vi "Tosca-Evaluate Input Event.vi"(0 "Progress In":T2, 1 "Event state in":T1, 7 "Term":refnum<class "Termination.lvclass">) -> (3 "Event state out":T1, 4 "Progress Out":T2, 8 "TTL condition true":bool)   [LabVIEW 2020]
uses:
  Typedefs/Tosca-Transition Progress.ctl
  Typedefs/Tosca-Trial Result Enum.ctl
  Typedefs/Tosca-TTL Event State.ctl
  Classes/Termination/Termination.lvclass
  Typedefs/Tosca-Termination Condition Action.ctl
  Classes/Termination/Termination.lvclass/Termination.ctl
  Classes/Termination/Read Input.vi
  Classes/Termination/Read Latency (ms).vi
  Classes/Termination/Read End after (ms).vi
  Classes/Termination/Read Action.vi
  Classes/Termination/Read Next.vi
  Classes/Termination/Read End on rep.vi
  Classes/Termination/Read Nttl.vi
  Classes/Termination/Read Tttl.vi
  Classes/Termination/Read Source.vi
  Classes/Termination/Read Result.vi
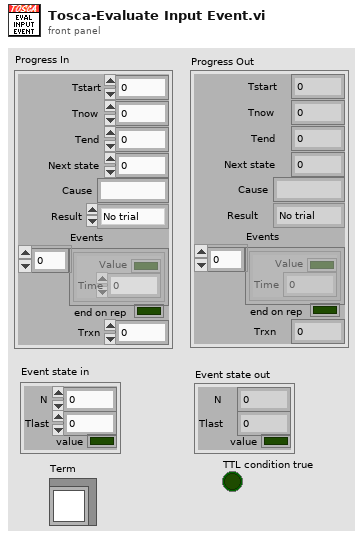
[diagram p1: front panel]
types:
  T1 = typedef "Tosca-TTL Event State.ctl" = cluster{"N":i32, "Tlast":dbl, "value":bool}
  T2 = typedef "Tosca-Transition Progress.ctl" = cluster{"Tstart":u32, "Tnow":u32, "Tend":dbl, "Next state":i32, "Cause":string, "Result":T3, "Events":cluster{"Value":bool, "Time":u32}[], "end on rep":bool, "Trxn":i32}
  T3 = typedef "Tosca-Trial Result Enum.ctl" = enum16{"No trial", "Go", "No go", "Error", "Abort"}
  T4 = typedef "Tosca-Termination Condition Action.ctl" = enum16{"End state", "Complete state", "TTL only"}
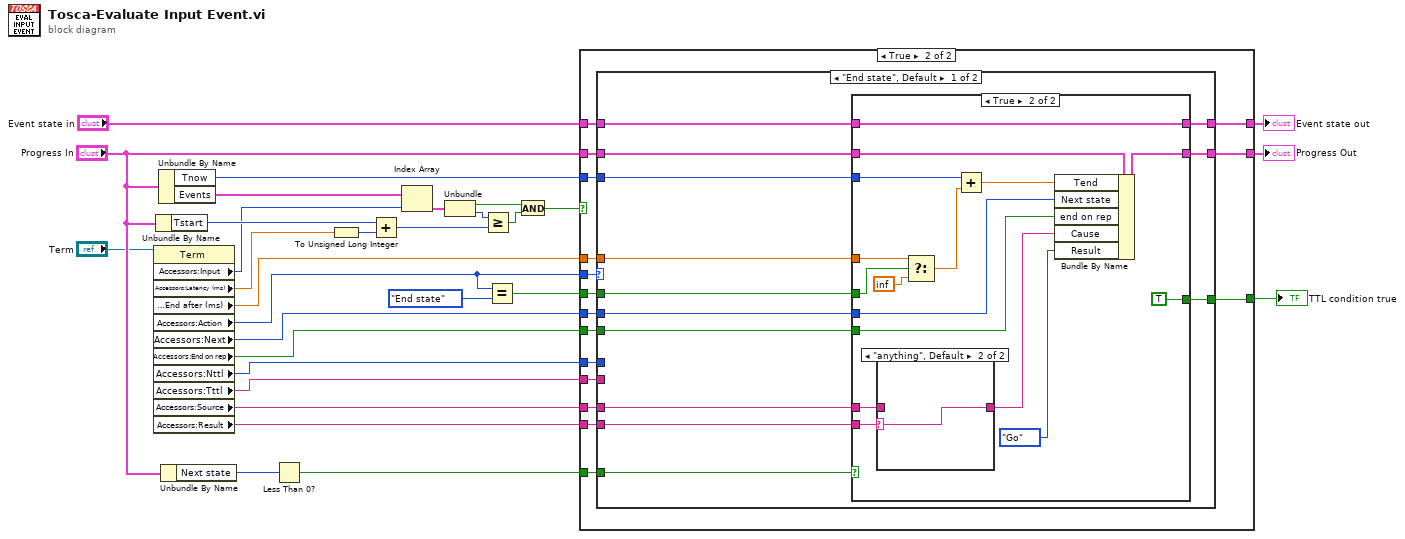
[diagram p0: block diagram]
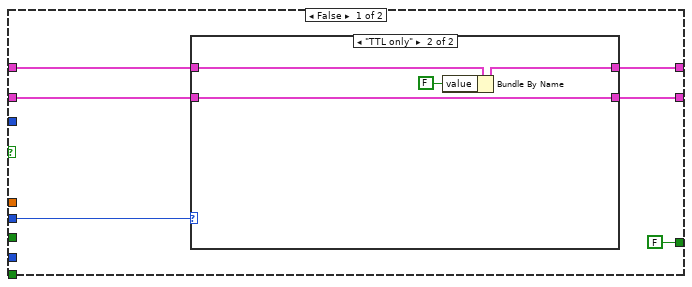
[diagram p2: hidden frame]
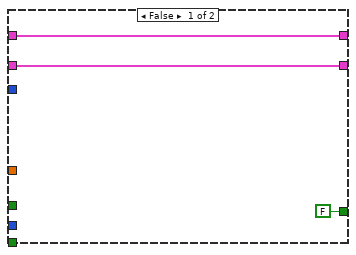
[diagram p4: hidden frame]
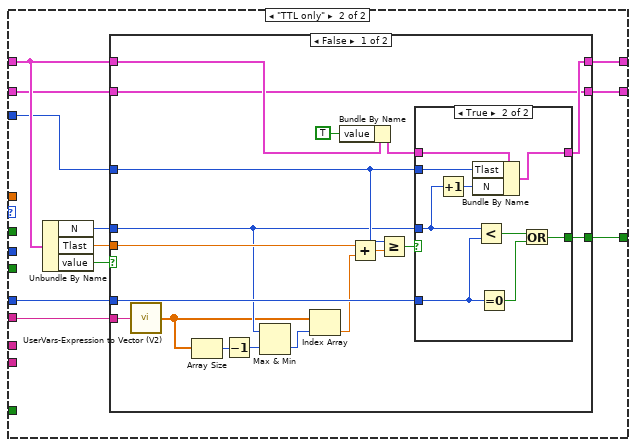
[diagram p6: hidden frame]
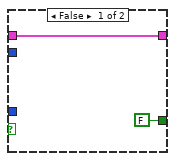
[diagram p7: hidden frame]
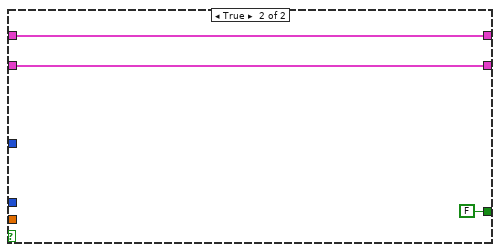
[diagram p8: hidden frame]
diagram:
  n1 = property class="Term"(reference="Term") -> ("Accessors:Input"=w1:i32, "Accessors:Latency (ms)"=w3:dbl, "Accessors:End after (ms)"=w4:dbl, "Accessors:Action"=w5:T4, "Accessors:Next"=w2:i32, "Accessors:End on rep"=w6:bool, "Accessors:Nttl"=w7:i32, "Accessors:Tttl"=w8:string, "Accessors:Source"=w9:string, "Accessors:Result"=w10:string)  [unwired: 1 in, 2 out]
  n2 = Unbundle By Name("Progress In") -> ("Tstart"=w20:u32)
  n3 = Unbundle By Name("Progress In") -> ("Tnow"=w23:u32, "Events"=w27:cluster{"Value":bool, "Time":u32}[])
  n4 = Unbundle By Name("Progress In") -> ("Next state"=w13:i32)
  n5 = Less Than 0?(x=w13) -> (x < 0?=w12:bool)
  n6 = To Unsigned Long Integer(number=w3) -> (unsigned 32bit integer=w21:u32)
  n7 = Add(x=w20, y=w21) -> (x+y=w22:u32)
  n8 = Index Array(array=w27, index=w1) -> (element=w30:cluster{"Value":bool, "Time":u32})
  n9 = Unbundle(w30) -> ("Value"=w26:bool, "Time"=w25:u32)
  n10 = Greater Or Equal?(x=w25, y=w22) -> (x >= y?=w28:bool)
  n11 = Equal?(x=w5, y=Tosca-Termination_Condition_Action."End state") -> (x = y?=w19:bool)
  n12 = And(x=w26, y=w28) -> (x .and. y?=w29:bool)
  n13 = case shown="True" w29 {
    tunnel: w4 -> [_ w57]
    tunnel: w19 -> [_ w58]
    tunnel: "Progress In" -> [w32 w56]
    tunnel: [w33 w53] -> w24
    tunnel: w10 -> [_ w55]
    tunnel: w9 -> [_ w54]
    tunnel: w2 -> [_ w52]
    tunnel: w6 -> [_ w51]
    tunnel: w23 -> [_ w50]
    tunnel: w5 -> [w31 w49]
    tunnel: [FALSE w48] -> w17
    tunnel: [w34 w47] -> w15
    tunnel: "Event state in" -> [w35 w46]
    tunnel: w7 -> [_ w45]
    tunnel: w8 -> [_ w44]
    tunnel: w12 -> [_ w43]
    frame False {
      n14 = case shown="\"TTL only\"" w31 {
        tunnel: w35 -> [w38 w42]
        tunnel: [w38 w40] -> w34
        tunnel: [w37 w41] -> w33
        tunnel: w32 -> [w37 w41]
        frame "End state", Default {
        }
        frame "TTL only" {
          n15 = Bundle By Name(cluster=w42, "value"=FALSE) -> (w40:T1)
        }
      }
    }
    frame True {
      n16 = case shown="\"End state\", Default" w49 {
        tunnel: w58 -> [w71 _]
        tunnel: w57 -> [w70 _]
        tunnel: w56 -> [w69 w95]
        tunnel: w55 -> [w68 _]
        tunnel: w54 -> [w67 _]
        tunnel: [w66 w94] -> w53
        tunnel: w52 -> [w65 _]
        tunnel: w51 -> [w64 _]
        tunnel: w50 -> [w63 w100]
        tunnel: [w62 w98] -> w48
        tunnel: [w61 w102] -> w47
        tunnel: w46 -> [w60 w103]
        tunnel: w45 -> [_ w99]
        tunnel: w44 -> [_ w97]
        tunnel: w43 -> [w59 _]
        frame "End state", Default {
          n17 = case shown="True" w59 {
            tunnel: w71 -> [_ w90]
            tunnel: w70 -> [_ w89]
            tunnel: w69 -> [w73 w87]
            tunnel: w68 -> [_ w86]
            tunnel: w67 -> [_ w85]
            tunnel: [w73 w84] -> w66
            tunnel: w65 -> [_ w82]
            tunnel: w64 -> [_ w81]
            tunnel: w63 -> [_ w80]
            tunnel: [FALSE TRUE] -> w62
            tunnel: [w74 w76] -> w61
            tunnel: w60 -> [w74 w76]
            frame False {
            }
            frame True {
              n18 = case shown="\"anything\", Default" w86 {
                selector: w86 -> [_ w92]
                tunnel: [w91 w92] -> w83
                tunnel: w85 -> [w91 _]
                frame "" {
                }
                frame "anything", Default {
                  # "Resp = CS+"
                }
              }
              n19 = Select(t=w89, s=w90, f=inf) -> (s? t:f=w79:dbl)
              n20 = Add(x=w80, y=w79) -> (x+y=w78:dbl)
              n21 = Bundle By Name(cluster=w87, "Tend"=w78, "Next state"=w82, "end on rep"=w81, "Cause"=w83, "Result"=Tosca-Trial_Result_Enum."Go") -> (w84:T2)
            }
          }
        }
        frame "TTL only" {
          n22 = Unbundle By Name(w103) -> ("N"=w96:i32, "Tlast"=w101:dbl, "value"=w93:bool)
          n23 = case shown="False" w93 {
            tunnel: w103 -> [w121 w134]
            tunnel: [w120 w134] -> w102
            tunnel: w101 -> [w119 _]
            tunnel: w100 -> [w117 _]
            tunnel: w99 -> [w115 _]
            tunnel: [w114 FALSE] -> w98
            tunnel: w97 -> [w113 _]
            tunnel: w96 -> [w110 _]
            tunnel: w95 -> [w106 w135]
            tunnel: [w106 w135] -> w94
            frame False {
              n24 = call "UserVars-Expression to Vector (V2).vi"("Expr"=w113) -> ("Values"=w109:dbl[])  [unwired: 13 in, 1 out]
              n25 = Array Size(array=w109) -> (size(s)=w112:i32)
              n26 = Decrement(x=w112) -> (x-1=w111:i32)
              n27 = Max & Min(x=w110, y=w111) -> (min(x,y)=w108:i32)  [unwired: 1 out]
              n28 = Index Array(array=w109, index=w108) -> (element=w107:dbl)
              n29 = Bundle By Name(cluster=w121, "value"=TRUE) -> (w105:T1)
              n30 = Add(x=w119, y=w107) -> (x+y=w118:dbl)
              n31 = Greater Or Equal?(x=w117, y=w118) -> (x >= y?=w116:bool)
              n32 = case shown="True" w116 {
                tunnel: w110 -> [_ w124]
                tunnel: w105 -> [w123 w131]
                tunnel: [w123 w130] -> w120
                tunnel: w117 -> [_ w129]
                tunnel: w115 -> [_ w126]
                tunnel: [FALSE w125] -> w114
                frame False {
                }
                frame True {
                  n33 = Increment(x=w124) -> (x+1=w132:i32)
                  n34 = Bundle By Name(cluster=w131, "Tlast"=w129, "N"=w132) -> (w130:T1)
                  n35 = Less?(x=w124, y=w126) -> (x < y?=w127:bool)
                  n36 = Equal To 0?(x=w126) -> (x = 0?=w128:bool)
                  n37 = Or(x=w127, y=w128) -> (x .or. y?=w125:bool)
                }
              }
            }
            frame True {
            }
          }
        }
      }
    }
  }
  "Progress Out" <- w24
  "TTL condition true" <- w17
  "Event state out" <- w15
